vi "PPFS_Test.vi"   [LabVIEW 2019]
doc: "This VI is called when test mode begins, and will automatically be terminated when it ends. You can add manual or automatic tests and invoke them from the dashboard."
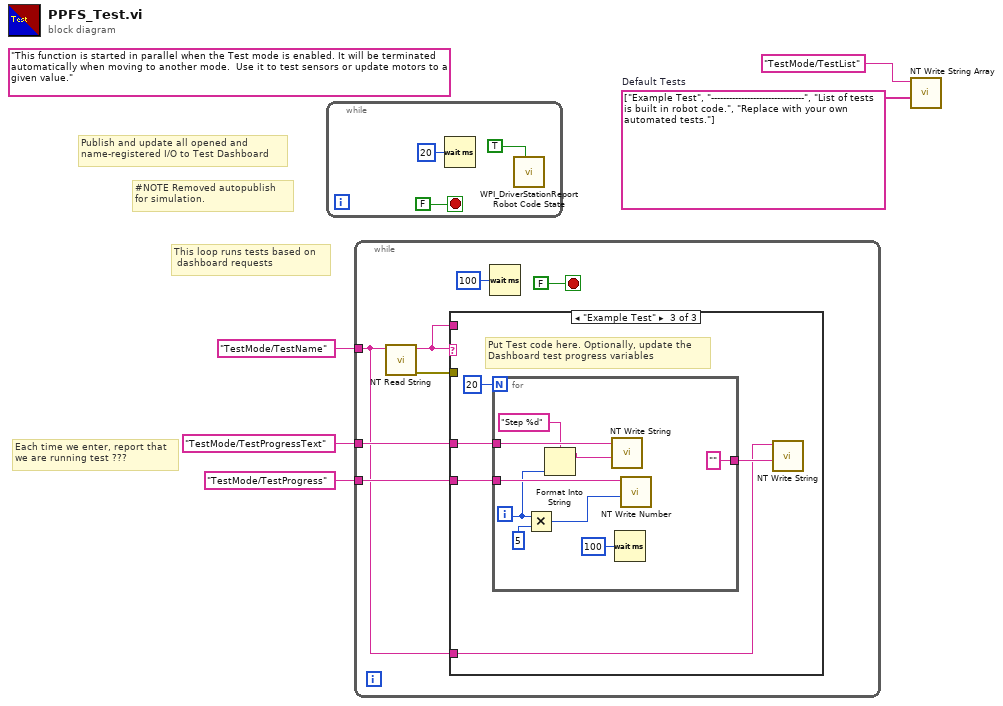
[diagram p0: block diagram]
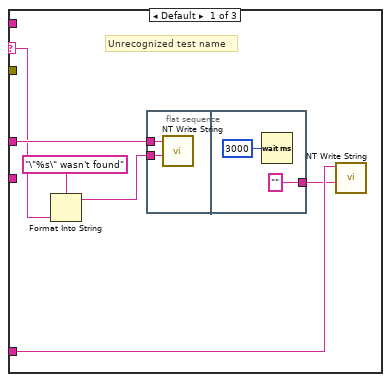
[diagram p2: hidden frame]
diagram:
  w2 = string[] ["Example Test", "-------------------------------", "List of tests is built in robot code.", "Replace with your own automated tests."]  # Default Tests
  (unwired) "This function is started in parallel when the Test mode is enabled. It will be terminated automatically when moving to another mode.  Use it to test sensors or update motors to a given value."
  # "#NOTE Removed autopublish\nfor simulation."
  # "This loop runs tests based on \n dashboard requests"
  # "Publish and update all opened and\nname-registered I/O to Test Dashboard"
  # "Each time we enter, report that\nwe are running test ???"
  n1 = while {
    stop <- FALSE stop-if-true
    n2 = Wait (ms)(milliseconds to wait=u32 20) -> ()  [unwired: 1 out]
    n3 = call <vilib>:"WPI_DriverStationReport Robot Code State.vi"("Test"=TRUE ("Autonomous")) -> ()  [unwired: 10 in, 1 out]
  }
  n4 = while {
    tunnel: "TestMode/TestName" ("Name") -> [w10]
    tunnel: "TestMode/TestProgressText" ("Name") -> [w13]
    tunnel: "TestMode/TestProgress" ("Name") -> [w12]
    stop <- FALSE stop-if-true
    n5 = call <vilib>:"NT Read String.vi"("name"=w10) -> ("error out"=w9:errorcluster, "value"=w11:string)  [unwired: 8 in, 1 out]
    n6 = case shown="\"Example Test\"" w11 {
      selector: w11 -> [w20 _ _]
      tunnel: w10 -> [w17 _ w26]
      tunnel: w13 -> [w21 _ w29]
      tunnel: w12 -> [_ _ w30]
      tunnel: w11 -> [_ _ _]
      tunnel: w9 -> [_ _ _]
      frame Default {
        # "Unrecognized test name"
        n7 = Format Into String(format string="\"%s\" wasn't found" ("Name"), w20) -> (resulting string=w19:string)  [unwired: 2 in, 1 out]
        n8 = flat-sequence {
          tunnel: w21 -> [w22]
          tunnel: w19 -> [w23]
          tunnel: ["" ("Name")] -> w16
          frame #0 {
            n9 = call <vilib>:"NT Write String.vi"("value"=w23, "name"=w22) -> ()  [unwired: 9 in, 1 out]
          }
          frame #1 {
            n10 = Wait (ms)(milliseconds to wait=u32 3000) -> ()  [unwired: 1 out]
          }
        }
        n11 = call <vilib>:"NT Write String.vi"("value"=w16, "name"=w17) -> ()  [unwired: 9 in, 1 out]
      }
      frame "" {
        # "No test to run"
      }
      frame "Example Test" {
        # "Put Test code here. Optionally, update the\nDashboard test progress variables"
        n12 = for {
          N: 20 -> [_]
          tunnel: w30 -> [w39]
          tunnel: w29 -> [w37]
          tunnel: ["" ("String")] -> w27
          i -> [w34]
          n13 = Multiply(x=w34, y=u32 5 ("milliseconds to wait")) -> (x*y=w35:u32)
          n14 = Format Into String(format string="Step %d", w34) -> (resulting string=w32:string)  [unwired: 2 in, 1 out]
          n15 = call <vilib>:"NT Write String.vi"("value"=w32, "name"=w37) -> ()  [unwired: 9 in, 1 out]
          n16 = Wait (ms)(milliseconds to wait=u32 100) -> ()  [unwired: 1 out]
          n17 = call <vilib>:"NT Write Number.vi"("value"=w35, "name"=w39) -> ()  [unwired: 9 in, 1 out]
        }
        n18 = call <vilib>:"NT Write String.vi"("value"=w27, "name"=w26) -> ()  [unwired: 9 in, 1 out]
      }
    }
    n19 = Wait (ms)(milliseconds to wait=u32 100) -> ()  [unwired: 1 out]
  }
  n20 = call <vilib>:"NT Write String Array.vi"("value"=w2, "name"="TestMode/TestList" ("Name")) -> ()  [unwired: 9 in, 1 out]
